vi "test_main_cam.vi"   [LabVIEW 2019]
uses:
  <vilib>/vision/driver/IMAQdx.llb/IMAQdx Buffer Number Mode.ctl
  <vilib>/vision/driver/NI_Vision_Acquisition_Software.lvlib
types:
  T1 = typedef "IMAQdx.ctl" = refnum<k21>
  T2 = typedef "IMAQ Image.ctl" = refnum<image>
  T3 = typedef "NI_Vision_Acquisition_Software.lvlib/IMAQdx Buffer Number Mode.ctl" = enum32{"Next", "Last", "Buffer Number", "Every", "Last New"}
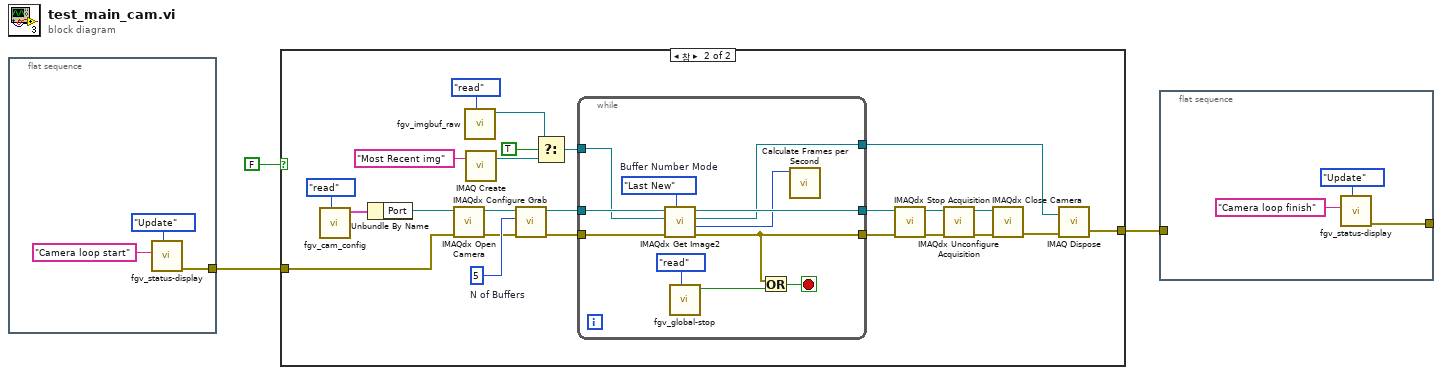
[diagram p0: block diagram]
diagram:
  n1 = flat-sequence {
    tunnel: [w4] -> w3
    frame #0 {
      n2 = call "fgv_status-display.vi"("Mode"=enum16{"Initial", "Update", "Clear"}."Update", "title"="Camera loop start" ("String in 1")) -> ("error out"=w4:errorcluster)  [unwired: 9 in]
    }
  }
  n3 = case shown="참" FALSE {
    tunnel: w3 -> [_ w13]
    tunnel: [_ w12] -> w2
    frame False {
    }
    frame True {
      w20 = u32 5  # N of Buffers
      n4 = call "fgv_cam_config.vi"("cmd"=enum16{"read", "write"}."read") -> ("camera cfg out"=w15:cluster{"Port":T1, "Camera file":path})  [unwired: 10 in]
      n5 = Unbundle By Name(w15) -> ("Port"=w14:T1)
      n6 = call <vilib>:"IMAQdx Open Camera.vi"("error in"=w13, "Session In"=w14) -> ("error out"=w19:errorcluster, "Session Out"=w21:T1)  [unwired: 1 in, 7 out]
      n7 = call "fgv_imgbuf_raw.vi"("cmd"=enum16{"create", "close", "write", "read"}."read") -> ("Image"=w9:T2)  [unwired: 9 in, 1 out]
      n8 = call "IMAQ Create"("Image Name"="Most Recent img") -> ("New Image"=w10:T2)  [unwired: 3 in, 2 out]
      n9 = call <vilib>:"IMAQdx Configure Grab.vi"("error in"=w19, "Number of Buffers"=w20, "Session In"=w21) -> ("error out"=w17:errorcluster, "Session Out"=w18:T1)  [unwired: 7 in]
      n10 = Select(t=w9, s=TRUE, f=w10) -> (s? t:f=w7:T2)
      n11 = while {
        tunnel: [w36] -> w29
        tunnel: w17 -> [w39]
        tunnel: w18 -> [w40]
        tunnel: [w34] -> w30
        tunnel: w7 -> [w38]
        tunnel: [w31] -> w22
        stop <- w41 stop-if-true
        w37 = IMAQdx_Buffer_Number_Mode."Last New"  # Buffer Number Mode
        n12 = call <vilib>:"IMAQdx Get Image2.vi"("Buffer Number Mode (Next)"=w37, "error in"=w39, "Image In"=w38, "Session In"=w40) -> ("error out"=w34:errorcluster, "Buffer Number Out"=w35:u32, "Image Out"=w31:T2, "Session Out"=w36:T1)  [unwired: 4 in]
        n13 = call "fgv_global-stop.vi"("cmd"=enum16{"init", "stop", "read"}."read") -> ("val_out"=w32:bool)  [unwired: 10 in]
        n14 = Or(x=w34, y=w32) -> (x .or. y?=w41:bool)
        n15 = call <vilib>:"Calculate Frames per Second.vi"("Buffer Number"=w35) -> ()  [unwired: 8 in, 3 out]
      }
      n16 = call <vilib>:"IMAQdx Stop Acquisition.vi"("error in"=w30, "Session In"=w29) -> ("error out"=w25:errorcluster, "Session Out"=w26:T1)  [unwired: 8 out]
      n17 = call <vilib>:"IMAQdx Unconfigure Acquisition.vi"("error in"=w25, "Session In"=w26) -> ("error out"=w28:errorcluster, "Session Out"=w27:T1)  [unwired: 8 out]
      n18 = call <vilib>:"IMAQdx Close Camera.vi"("error in"=w28, "Session In"=w27) -> ("error out"=w24:errorcluster)  [unwired: 9 out]
      n19 = call "IMAQ Dispose"("Image"=w22, "error in (no error)"=w24) -> ("error out"=w12:errorcluster)  [unwired: 4 in]
    }
  }
  n20 = flat-sequence {
    tunnel: w2 -> [_]
    tunnel: [w42] -> _
    frame #0 {
      n21 = call "fgv_status-display.vi"("Mode"=enum16{"Initial", "Update", "Clear"}."Update", "title"="Camera loop finish" ("String in 1")) -> ("error out"=w42:errorcluster)  [unwired: 9 in]
    }
  }
